vi "FTW-Logger-Process.vi"(0 "FTW Logger Configuration":string, 11 "error in":errorcluster) -> (15 "error out":errorcluster)   [LabVIEW 2013, in "FTW-Logger-Core.lvclass"]
uses:
  FTW-Logger-Core.lvclass
  FTW-Logger-Core.lvclass/FTW-Logger-Core.ctl
  Instance/FTW-ActorInstance.lvclass/FTW-ActorInstance.ctl
  JobSequencer/FTW-SEQ-Current.vi
  FTW-Logger.lvclass
  Message/Request/FTW-Message-IncomingRequest.lvclass
  Instance/FTW-ActorInstance.lvclass
panel:
  # "Inputs"
  # "Outputs"
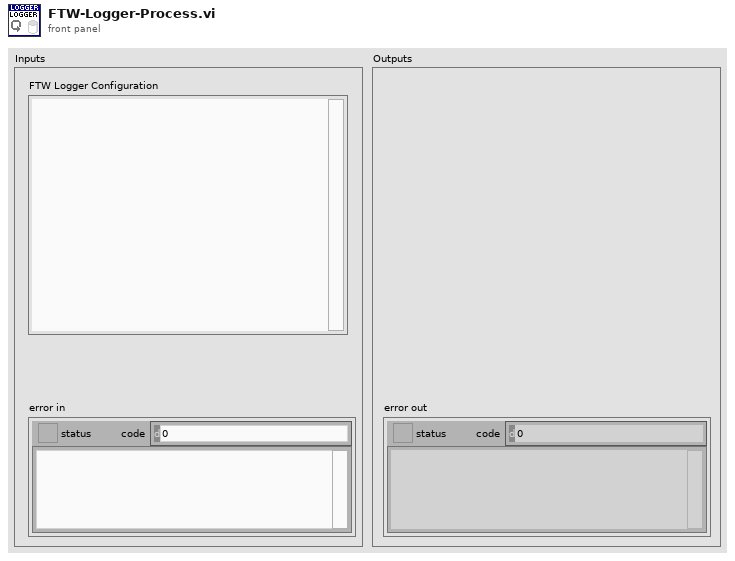
[diagram p1: front panel]
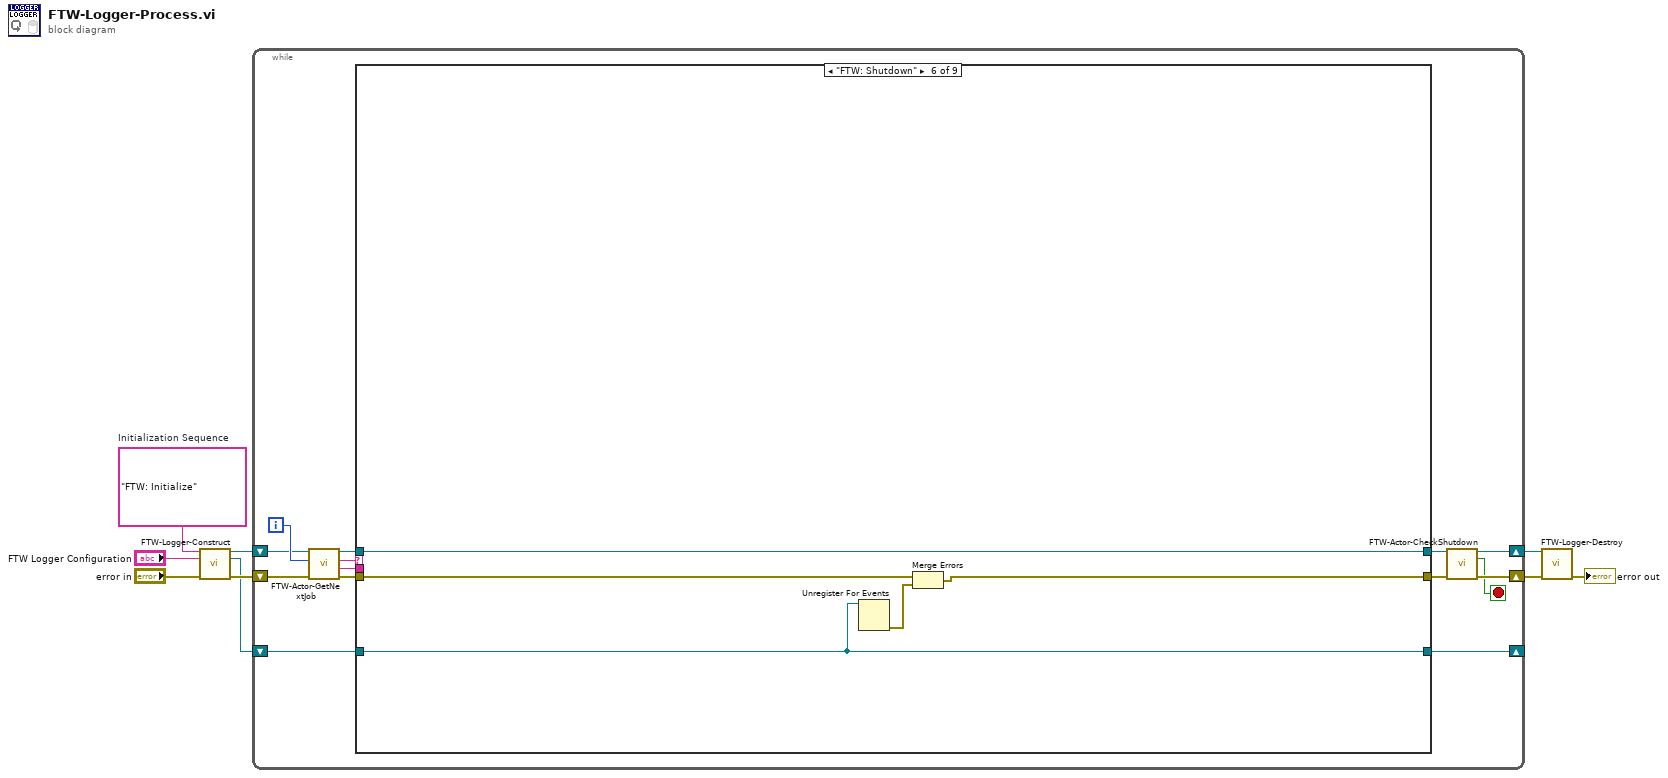
[diagram p0: block diagram]
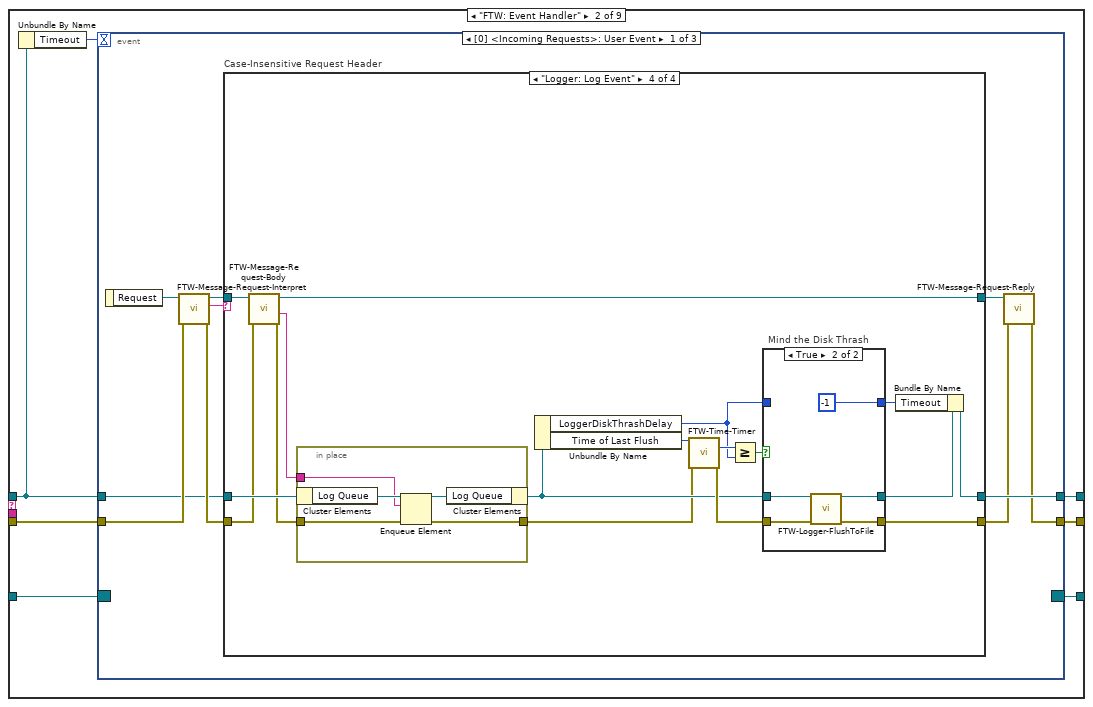
[diagram p3: hidden frame]
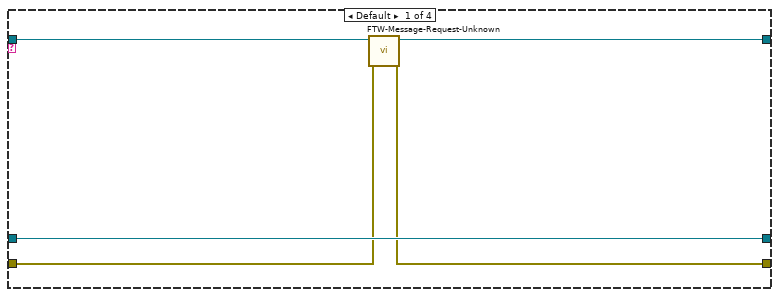
[diagram p4: hidden frame]
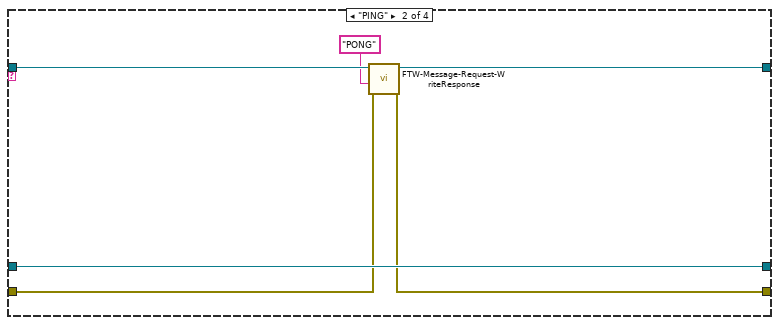
[diagram p5: hidden frame]
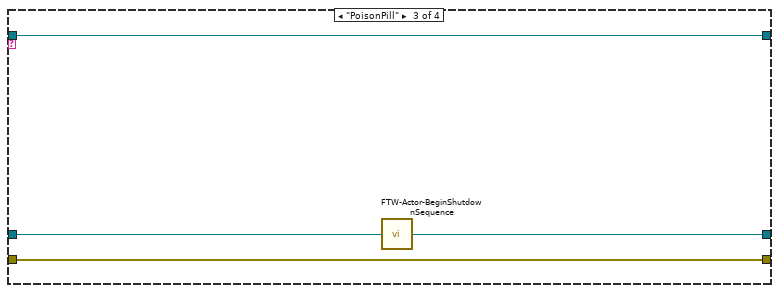
[diagram p6: hidden frame]
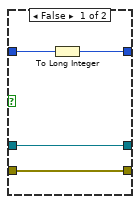
[diagram p7: hidden frame]
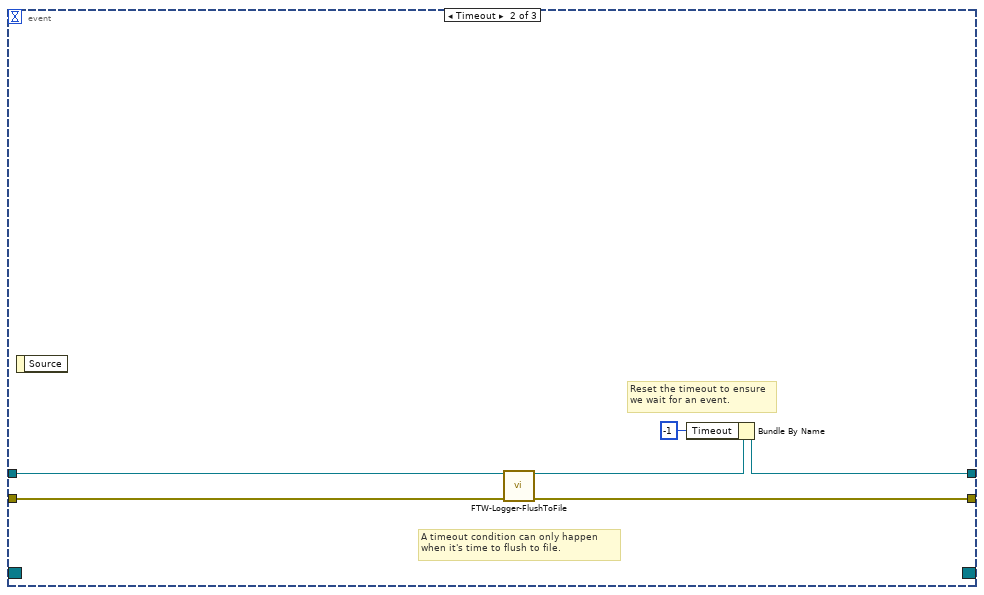
[diagram p8: hidden frame]
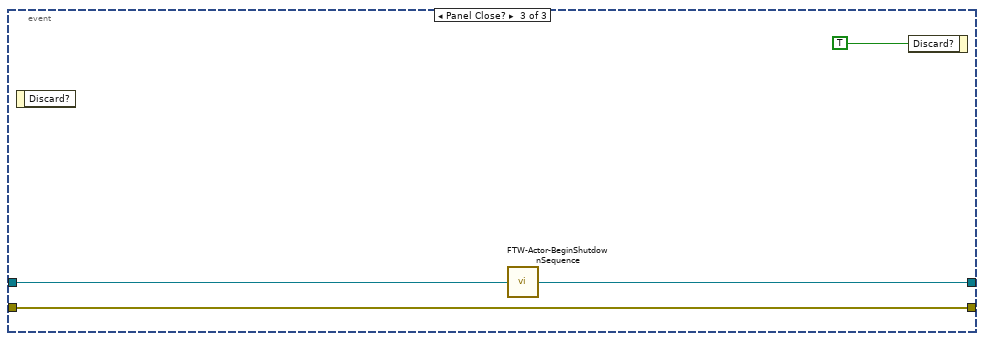
[diagram p9: hidden frame]
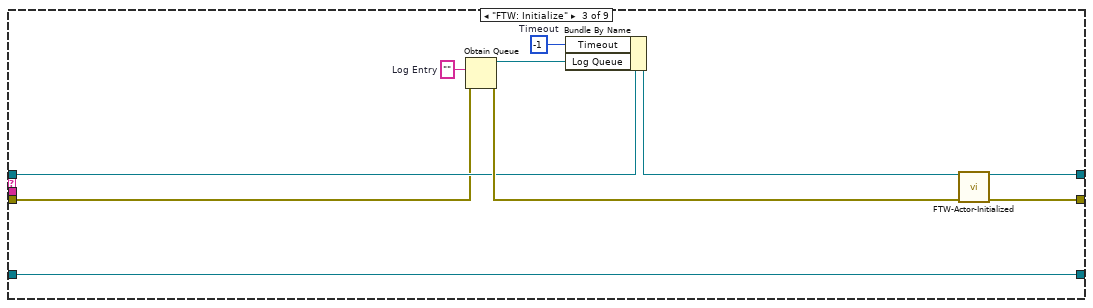
[diagram p10: hidden frame]
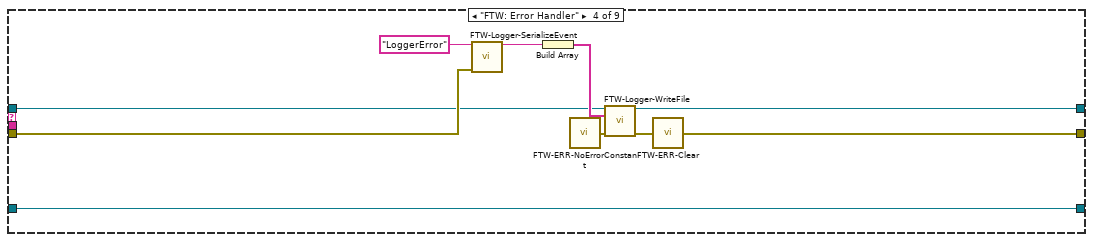
[diagram p11: hidden frame]
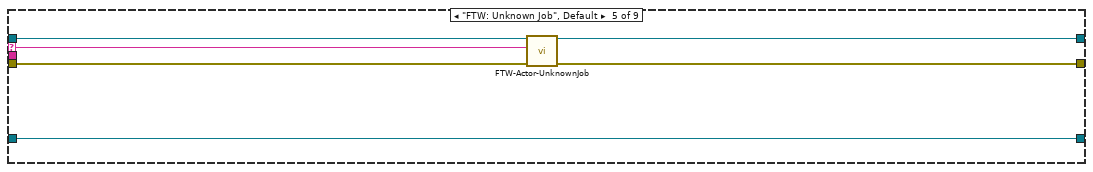
[diagram p12: hidden frame]
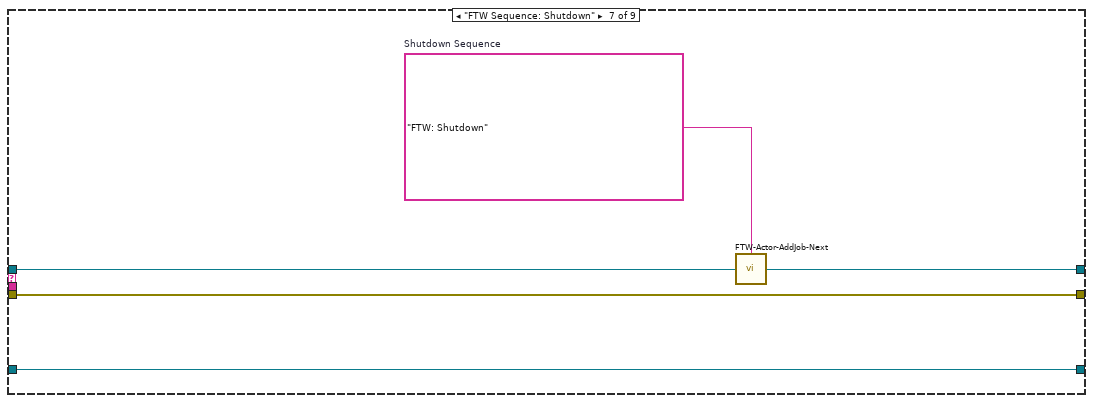
[diagram p13: hidden frame]
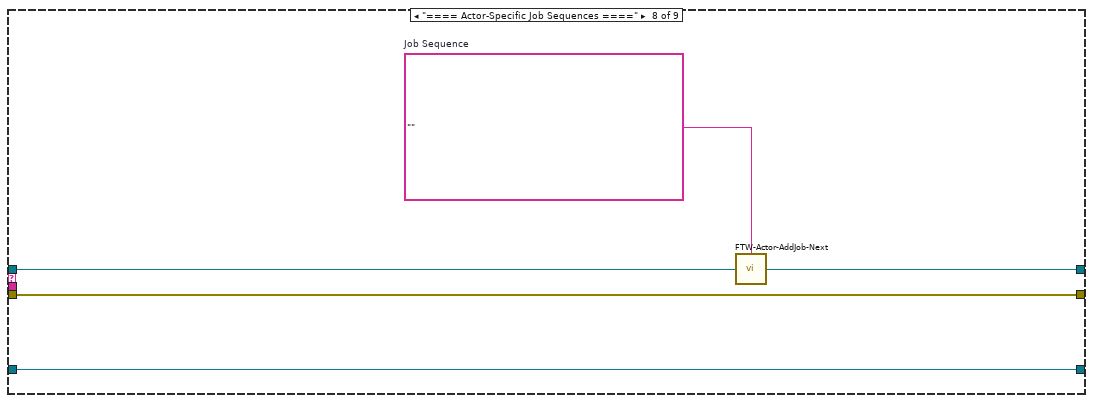
[diagram p14: hidden frame]
diagram:
  w2 = "FTW: Initialize"  # Initialization Sequence
  n1 = call "FTW-Logger-Construct.vi"("Initialization Sequence"=w2, "Logger Configuration"="FTW Logger Configuration", "error in"="error in") -> ("FTW Logger"=w6:refnum<class "FTW-Logger-Core.lvclass">, "Incoming Requests"=w3:refnum<event-registration>, "error out"=w5:errorcluster)  [unwired: 10 in]
  n2 = while {
    shift-right: [w12] -> w8
    shift-left: w5 -> [w21]
    shift-right: [w22] -> _
    shift-left: w3 -> [w23]
    shift-right: [w11] -> w9
    shift-left: w6 -> [w18]
    i -> [w20]
    stop <- w10 stop-if-true
    n3 = call "FTW-Actor-GetNextJob.vi"("error in"=w21, "Jobs Performed"=w20, "FTW Actor Instance"=w18) -> ("error out"=w19:errorcluster, "Job Data"=w15:string, "Job Name"=w16:string, "FTW Actor Instance out"=w17:refnum<class "FTW-Logger-Core.lvclass">)  [unwired: 5 in]
    n4 = case shown="\"FTW: Shutdown\"" w16 {
      selector: w16 -> [_ _ _ _ w121 _ _ _ _]
      tunnel: [w25 w33 w105 w115 w122 w130 w134 w139 w143] -> w13
      tunnel: w19 -> [w25 w32 w100 w117 w120 w127 w134 w139 w143]
      tunnel: w23 -> [w26 w31 w108 w119 w125 w128 w135 w140 w142]
      tunnel: [w26 w30 w108 w119 w125 w128 w135 w140 w142] -> w22
      tunnel: w17 -> [w24 w27 w101 w111 w124 w126 w132 w137 w141]
      tunnel: [w24 w28 w106 w112 w123 w126 w131 w136 w141] -> w14
      tunnel: w15 -> [_ _ _ _ _ _ _ _ _]
      frame "==== Featherweight Framework Jobs ====" {
      }
      frame "FTW: Event Handler" {
        n5 = Unbundle By Name(w27) -> ("Timeout"=w29:i32)
        n6 = event shown="[0] <Incoming Requests>: User Event" {
          selector: w31 -> [_ _ _]
          dyn-events: [_ _ _] -> w30
          timeout: w29 -> [_ _ _]
          tunnel: [w34 w94 w98] -> w33
          tunnel: w32 -> [w42 w95 w98]
          tunnel: [w41 w90 w96] -> w28
          tunnel: w27 -> [w40 w93 w97]
          event User Event {
            n7 = event-data() -> ("Request"=w38:refnum<class "FTW-Message-IncomingRequest.lvclass">)  [unwired: 1 in]
            n8 = call "FTW-Message-Request-Interpret.vi"("error in"=w42, "FTW Incoming Request"=w38) -> ("error out"=w43:errorcluster, "Request Header"=w39:string, "FTW Incoming Request out"=w37:refnum<class "FTW-Message-IncomingRequest.lvclass">)  [unwired: 7 in]
            n9 = case "Case-Insensitive Request Header" shown="\"Logger: Log Event\"" w39 {
              tunnel: [w45 w52 w58 w72] -> w35
              tunnel: w43 -> [w46 w53 w58 w65]
              tunnel: [w48 w54 w56 w68] -> w41
              tunnel: w40 -> [w48 w54 w57 w67]
              tunnel: w37 -> [w47 w51 w55 w61]
              tunnel: [w44 w49 w55 w60] -> w36
              frame Default {
                n10 = call "FTW-Message-Request-Unknown.vi"("error in"=w46, "FTW Incoming Request"=w47) -> ("error out"=w45:errorcluster, "FTW Incoming Request Out"=w44:refnum<class "FTW-Message-IncomingRequest.lvclass">)  [unwired: 8 in]
              }
              frame "PING" {
                n11 = call "FTW-Message-Request-WriteResponse.vi"("error in"=w53, "Response Body"="PONG" ("Response Header"), "FTW Incoming Request"=w51) -> ("error out"=w52:errorcluster, "FTW Incoming Request out"=w49:refnum<class "FTW-Message-IncomingRequest.lvclass">)  [unwired: 7 in]
              }
              frame "PoisonPill" {
                n12 = call "FTW-Actor-BeginShutdownSequence.vi"("FTW Actor Instance"=w57) -> ("FTW Actor Instance out"=w56:refnum<class "FTW-Logger-Core.lvclass">)  [unwired: 3 in]
              }
              frame "Logger: Log Event" {
                n13 = call "FTW-Message-Request-Body.vi"("error in"=w65, "FTW Incoming Request"=w61) -> ("error out"=w62:errorcluster, "Request Body"=w59:string, "FTW Incoming Request out"=w60:refnum<class "FTW-Message-IncomingRequest.lvclass">)  [unwired: 7 in]
                n14 = in-place {
                  in-place-border: w62 -> [w80]
                  in-place-border: [w77] -> w64
                  in-place-border: w59 -> [w76]
                  n15 = in-place-cluster #1(w67) -> ("Log Queue"=w79:refnum<queue>)
                  n16 = Enqueue Element(queue=w79, element=w76, error in (no error)=w80) -> (queue out=w78:refnum<queue>, error out=w77:errorcluster)  [unwired: 1 in, 1 out]
                  n17 = in-place-cluster #1("Log Queue"=w78) -> (w66:refnum<class "FTW-Logger-Core.lvclass">)
                }
                n18 = Unbundle By Name(w66) -> ("LoggerDiskThrashDelay"=w63:u32, "Time of Last Flush"=w75:u32)
                n19 = call "FTW-Time-Timer.vi"("Initial Tick Count"=w75, "error in"=w64) -> ("Elapsed Time"=w74:u32, "error out"=w73:errorcluster)  [unwired: 11 in, 1 out]
                n20 = Greater Or Equal?(x=w74, y=w63) -> (x >= y?=w71:bool)
                n21 = case "Mind the Disk Thrash" shown="True" w71 {
                  tunnel: [w84 w86] -> w69
                  tunnel: w66 -> [w84 w87]
                  tunnel: w73 -> [w83 w89]
                  tunnel: [w83 w88] -> w72
                  tunnel: [w81 -1 ("Timeout")] -> w70
                  tunnel: w63 -> [w82 _]
                  frame False {
                    n22 = To Long Integer(number=w82) -> (32bit integer=w81:i32)
                  }
                  frame True {
                    n23 = call "FTW-Logger-FlushToFile.vi"("FTW Logger"=w87, "error in"=w89) -> ("FTW Logger out"=w86:refnum<class "FTW-Logger-Core.lvclass">, "error out"=w88:errorcluster)  [unwired: 12 in]
                  }
                }
                n24 = Bundle By Name(cluster=w69, "Timeout"=w70) -> (w68:refnum<class "FTW-Logger-Core.lvclass">)
              }
            }
            n25 = call "FTW-Message-Request-Reply.vi"("error in"=w35, "FTW Incoming Request"=w36) -> ("error out"=w34:errorcluster)  [unwired: 8 in, 1 out]
          }
          event Timeout {
            # "Reset the timeout to ensure\nwe wait for an event."
            # "A timeout condition can only happen\nwhen it's time to flush to file."
            n26 = event-data() -> ()  [unwired: 1 in, 1 out]
            n27 = call "FTW-Logger-FlushToFile.vi"("FTW Logger"=w93, "error in"=w95) -> ("FTW Logger out"=w91:refnum<class "FTW-Logger-Core.lvclass">, "error out"=w94:errorcluster)  [unwired: 12 in]
            n28 = Bundle By Name(cluster=w91, "Timeout"=-1) -> (w90:refnum<class "FTW-Logger-Core.lvclass">)
          }
          event Panel Close? {
            n29 = event-data() -> ()  [unwired: 1 in, 1 out]
            n30 = call "FTW-Actor-BeginShutdownSequence.vi"("FTW Actor Instance"=w97) -> ("FTW Actor Instance out"=w96:refnum<class "FTW-Logger-Core.lvclass">)  [unwired: 3 in]
            n31 = event-data("Discard?"=TRUE) -> ()  [unwired: 1 in, 1 out]
          }
        }
      }
      frame "FTW: Initialize" {
        w102 = ""  # Log Entry
        w109 = -1  # Timeout
        n32 = Obtain Queue(element data type=w102, error in (no error)=w100) -> (queue out=w104:refnum<queue>, error out=w103:errorcluster)  [unwired: 3 in, 1 out]
        n33 = Bundle By Name(cluster=w101, "Timeout"=w109, "Log Queue"=w104) -> (w107:refnum<class "FTW-Logger-Core.lvclass">)
        n34 = call-dynamic "FTW-Actor-Initialized.vi"("FTW Actor Instance"=w107, "error in"=w103) -> ("FTW Actor Instance out"=w106:refnum<class "FTW-Logger-Core.lvclass">, "error out"=w105:errorcluster)  [unwired: 12 in]
      }
      frame "FTW: Error Handler" {
        n35 = call "FTW-Logger-SerializeEvent.vi"("Event Type"="LoggerError", "Error to Log"=w117) -> ("Serialized Event"=w114:string)  [unwired: 13 in]
        n36 = Build Array(w114) -> (w113:string[])
        n37 = call "FTW-ERR-NoErrorConstant.vi"() -> ("no error"=w110:errorcluster)
        n38 = call "FTW-Logger-WriteFile.vi"("FTW Logger"=w111, "Entries to Log"=w113, "error in"=w110) -> ("FTW Logger out"=w112:refnum<class "FTW-Logger-Core.lvclass">, "error out"=w116:errorcluster)  [unwired: 11 in]
        n39 = call "FTW-ERR-Clear.vi"("error to snuff"=w116) -> ("no error"=w115:errorcluster)
      }
      frame "FTW: Unknown Job", Default {
        n40 = call-dynamic "FTW-Actor-UnknownJob.vi"("FTW Actor Instance"=w124, "Unknown Job"=w121, "error in"=w120) -> ("FTW Actor Instance out"=w123:refnum<class "FTW-Logger-Core.lvclass">, "error out"=w122:errorcluster)  [unwired: 11 in]
      }
      frame "FTW: Shutdown" {
        n41 = Unregister For Events(event registration refnum=w128) -> (error out=w129:errorcluster)  [unwired: 1 in]
        n42 = Merge Errors(w127, w129) -> (w130:errorcluster)
      }
      frame "FTW Sequence: Shutdown" {
        w133 = "FTW: Shutdown"  # Shutdown Sequence
        n43 = call "FTW-Actor-AddJob-Next.vi"("Add Next in Job Queue"=w133, "FTW Actor Instance"=w132) -> ("FTW Actor Instance out"=w131:refnum<class "FTW-Logger-Core.lvclass">)  [unwired: 2 in]
      }
      frame "==== Actor-Specific Job Sequences ====" {
        w138 = ""  # Job Sequence
        n44 = call "FTW-Actor-AddJob-Next.vi"("Add Next in Job Queue"=w138, "FTW Actor Instance"=w137) -> ("FTW Actor Instance out"=w136:refnum<class "FTW-Logger-Core.lvclass">)  [unwired: 2 in]
      }
      frame "==== Actor-Specific Jobs ====" {
      }
    }
    n45 = call "FTW-Actor-CheckShutdown.vi"("FTW Actor Instance"=w14, "error in"=w13) -> ("FTW Actor Instance out"=w11:refnum<class "FTW-Logger-Core.lvclass">, "Shutdown?"=w10:bool, "error out"=w12:errorcluster)  [unwired: 11 in]
  }
  n46 = call "FTW-Logger-Destroy.vi"("FTW Logger"=w9, "error in"=w8) -> ("error out"=→"error out":errorcluster)  [unwired: 13 in]
